vi "SubPanel_DataCollection_Rev11_v4.vi"(0 "DCPowerInformationClusterArray_Input":T6(array[cluster]), 1 "VISAPowerInfoInputArray":T11(array[cluster]), 2 "Run Data SubPanel Input":T10, 3 "RF Block Parameters":T9, 4 "Oscilloscope Info Array":T8(array[cluster]) {"vertical coupling" items=["AC", "DC", "Ground"]}, 6 "New Run?":bool, 7 "error in":errorcluster) -> (10 "data iterating in loop":T2(array[cluster]), 12 "each channel cluster":T2(array[cluster]), 13 "Array of all channels?":dbl[][](array[numeric]), 14 "all channel clusters as a large array":T1(array[cluster]), 16 "data going into the binary file":T3, 20 "DCPowerInformationClusterArray_Output":T6(array[cluster]), 21 "VISAPowerInfoInputOutput":T11(array[cluster]), 22 "Run Data SubPanel Output":T10, 23 "RF Block Parameters Output":T9, 24 "Oscilloscope Info Array Output":T8(array[cluster]) {"vertical coupling" items=["AC", "DC", "Ground"]}, 25 "Reinitialize?":bool, 26 "Data Was Collected?":bool, 27 "error out":errorcluster)   [LabVIEW 2019]
uses:
  Controls/QueueDataControl.ctl
  Controls/DataBlockControl.ctl
  Controls/QueueDataControl_V2.ctl
  <vilib>/Analysis/NI_AALBase.lvlib
  Controls/QueueDataControl_V3.ctl
  <vilib>/Utility/file.llb/Write Delimited Spreadsheet (DBL).vi
  <vilib>/Analysis/1siggen.llb/Ramp Pattern by Delta.vi
  Controls/RFBlockControl.ctl
  <instrlib>/niScope/Controls/niScope vertical coupling.ctl
panel:
  out "supplemental datafile concatenated":i32[](array[numeric])
  out "supplemental datafile array":i32[][](array[numeric])
  out "supplemental datafile":i32[](array[numeric])
  out "datafile in array":T4[][](array[typedef])
  out "datafile in concatenation":T4[](array[typedef])
  out "datafile in loop":T4[](array[typedef])
  out "output cluster 2":T5
  out "Array":dbl[][][](array[numeric])
  out "DCPowerInformationClusterArray_Input 2":T6(array[cluster])
  out "Exiting":bool
  out "output cluster":T5
  out "Full Run Information":string
  out "Ready For Next Run?":bool
  in  "Next Run":bool
  out "Latchup Output Data":dbl[][](array[numeric])
  out "Recording Data":bool
  out "Current 2":waveform(dbl)[](graph)
  out "Voltage 2":waveform(dbl)[](graph)
  out "Current":waveform(dbl)[](graph)
  out "Voltage":waveform(dbl)[](graph)
  in  "End Collecting":bool
  in  "Record Data Toggle":bool
  out "error of collection":errorcluster
  in  "force exit SubVI":bool
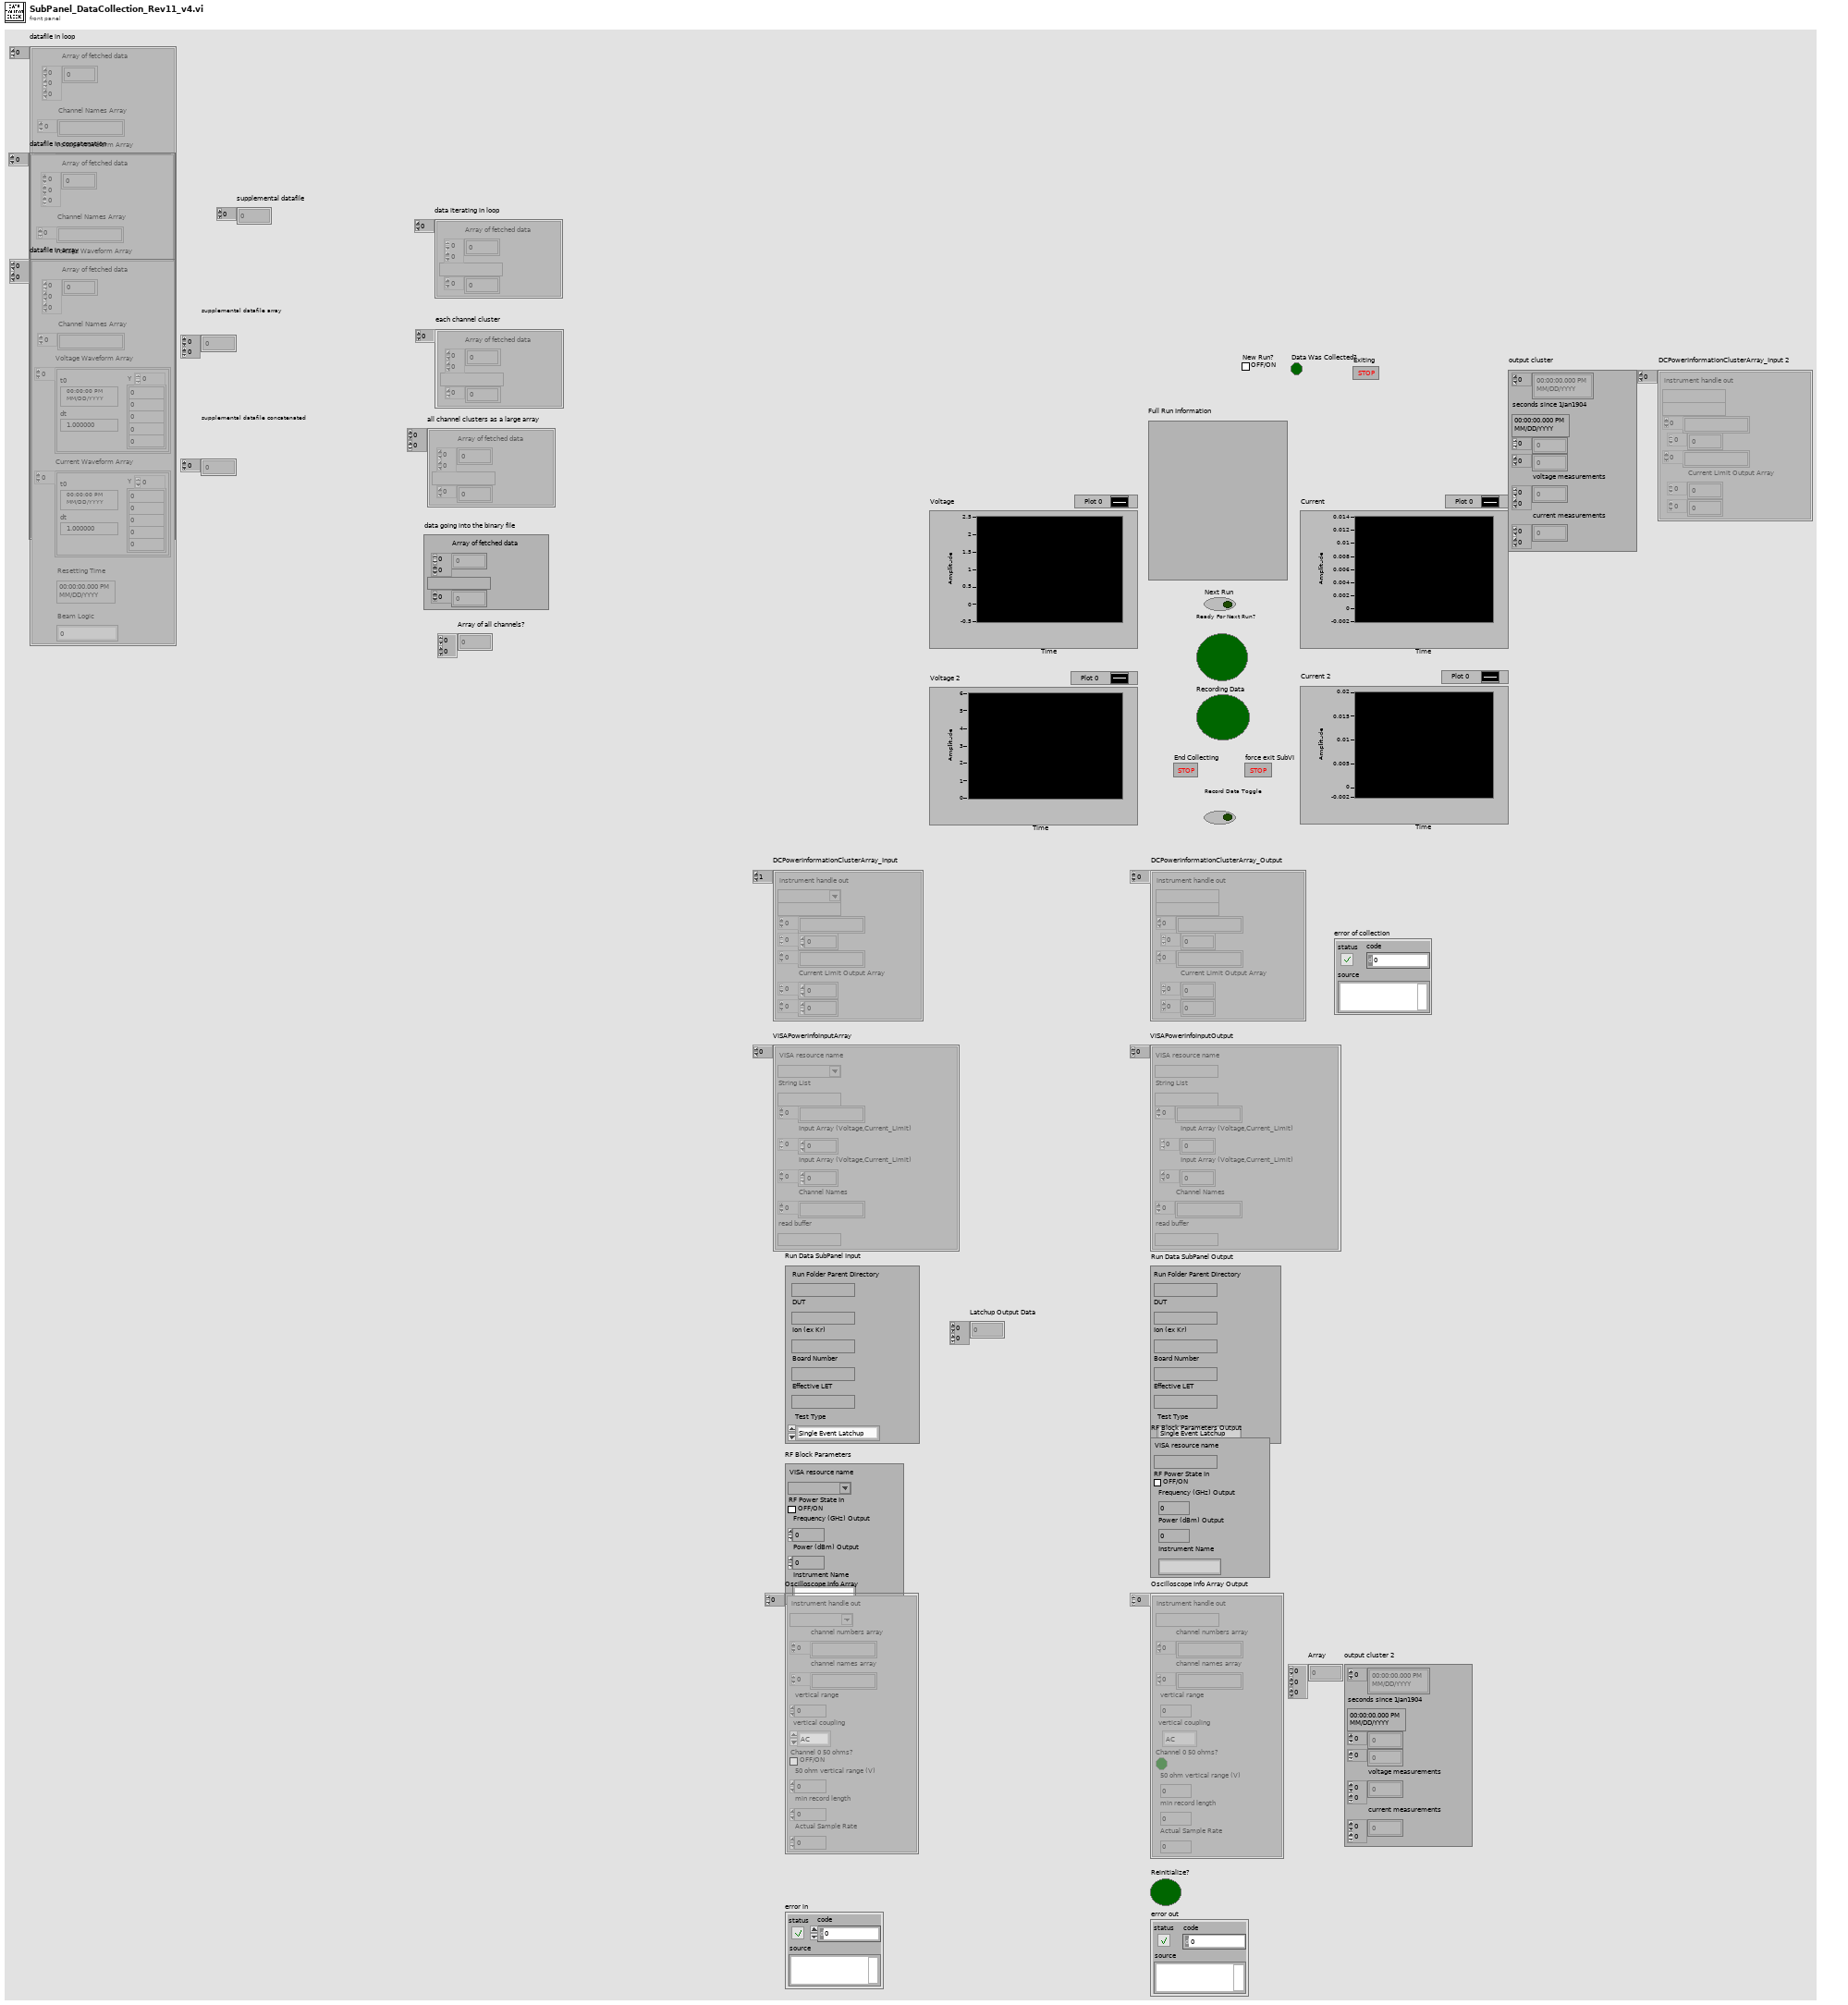
[diagram p1: front panel]
types:
  T1 = cluster{"Array of fetched data":dbl[][], string, i32[]}[][]
  T2 = cluster{"Array of fetched data":dbl[][], string, i32[]}[]
  T3 = cluster{"Array of fetched data":dbl[][], string, i32[]}
  T4 = typedef "QueueDataControl_V3.ctl" = cluster{"Array of fetched data":dbl[][][], "Channel Names Array":string[], "Voltage Waveform Array":waveform(dbl)[], "Current Waveform Array":waveform(dbl)[], "Resetting Time":timestamp, "Beam Logic":dbl}
  T5 = cluster{timestamp[], "seconds since 1Jan1904":timestamp, dbl[], i32[], "voltage measurements":dbl[][], "current measurements":dbl[][]}
  T6 = cluster{"instrument handle out":refnum<k15>, string, string[], dbl[], string[], "Current Limit Output Array":dbl[], dbl[]}[]
  T7 = typedef "niScope vertical coupling.ctl" = i32
  T8 = cluster{"instrument handle out":refnum<k15>, "channel numbers array":string[], "channel names array":string[], "vertical range":dbl, "vertical coupling":T7, "Channel 0 50 ohms?":bool, "50 ohm vertical range (V)":dbl, "min record length":i32, "Actual Sample Rate":dbl}[]
  T9 = typedef "RFBlockControl.ctl" = cluster{"VISA resource name":refnum<visa-resource-name>, "RF Power State In":bool, "Frequency (GHz) Output":dbl, "Power (dBm) Output":dbl, "Instrument Name":string}
  T10 = typedef "DataBlockControl.ctl" = cluster{"Run Folder Parent Directory":path, "DUT":string, "Ion (ex Kr)":string, "Board Number":string, "Effective LET":string, "Test Type":enum16{"Single Event Latchup", "Single Event Transient", "Single Event Upset"}}
  T11 = cluster{"VISA resource name":refnum<visa-resource-name>, "String List":string, string[], "Input Array (Voltage,Current_Limit)":dbl[], "Input Array (Voltage,Current_Limit)":dbl[], "Channel Names":string[], "read buffer":string}[]
  T12 = typedef "QueueDataControl_V2.ctl" = cluster{"Time Stamp Array":timestamp[], "Initial Time":timestamp, "dt measurement array":dbl[], "samples per capture":i32[], "voltage measurements":dbl[][], "current measurements":dbl[][]}
  T13 = cluster{"IVI Refnum out":refnum<k15>, string, "voltage level channel 23":dbl, "Channel Name 23":string, "Current Limit":dbl, "Measure Record dt":dbl, string}[]
  T14 = typedef "QueueDataControl.ctl" = cluster{"Rolling Timer":timestamp, "Initial Time":timestamp, "dt between samples":dbl[], "number of samples per fetch":i32[], "voltage measurements":dbl[][], "current measurements":dbl[][]}
  T15 = enum16{"big-endian, network order", "native, host order", "little-endian"}
  T16 = enum16{"open", "replace", "create", "open or create", "replace or create", "replace or create with confirmation"}
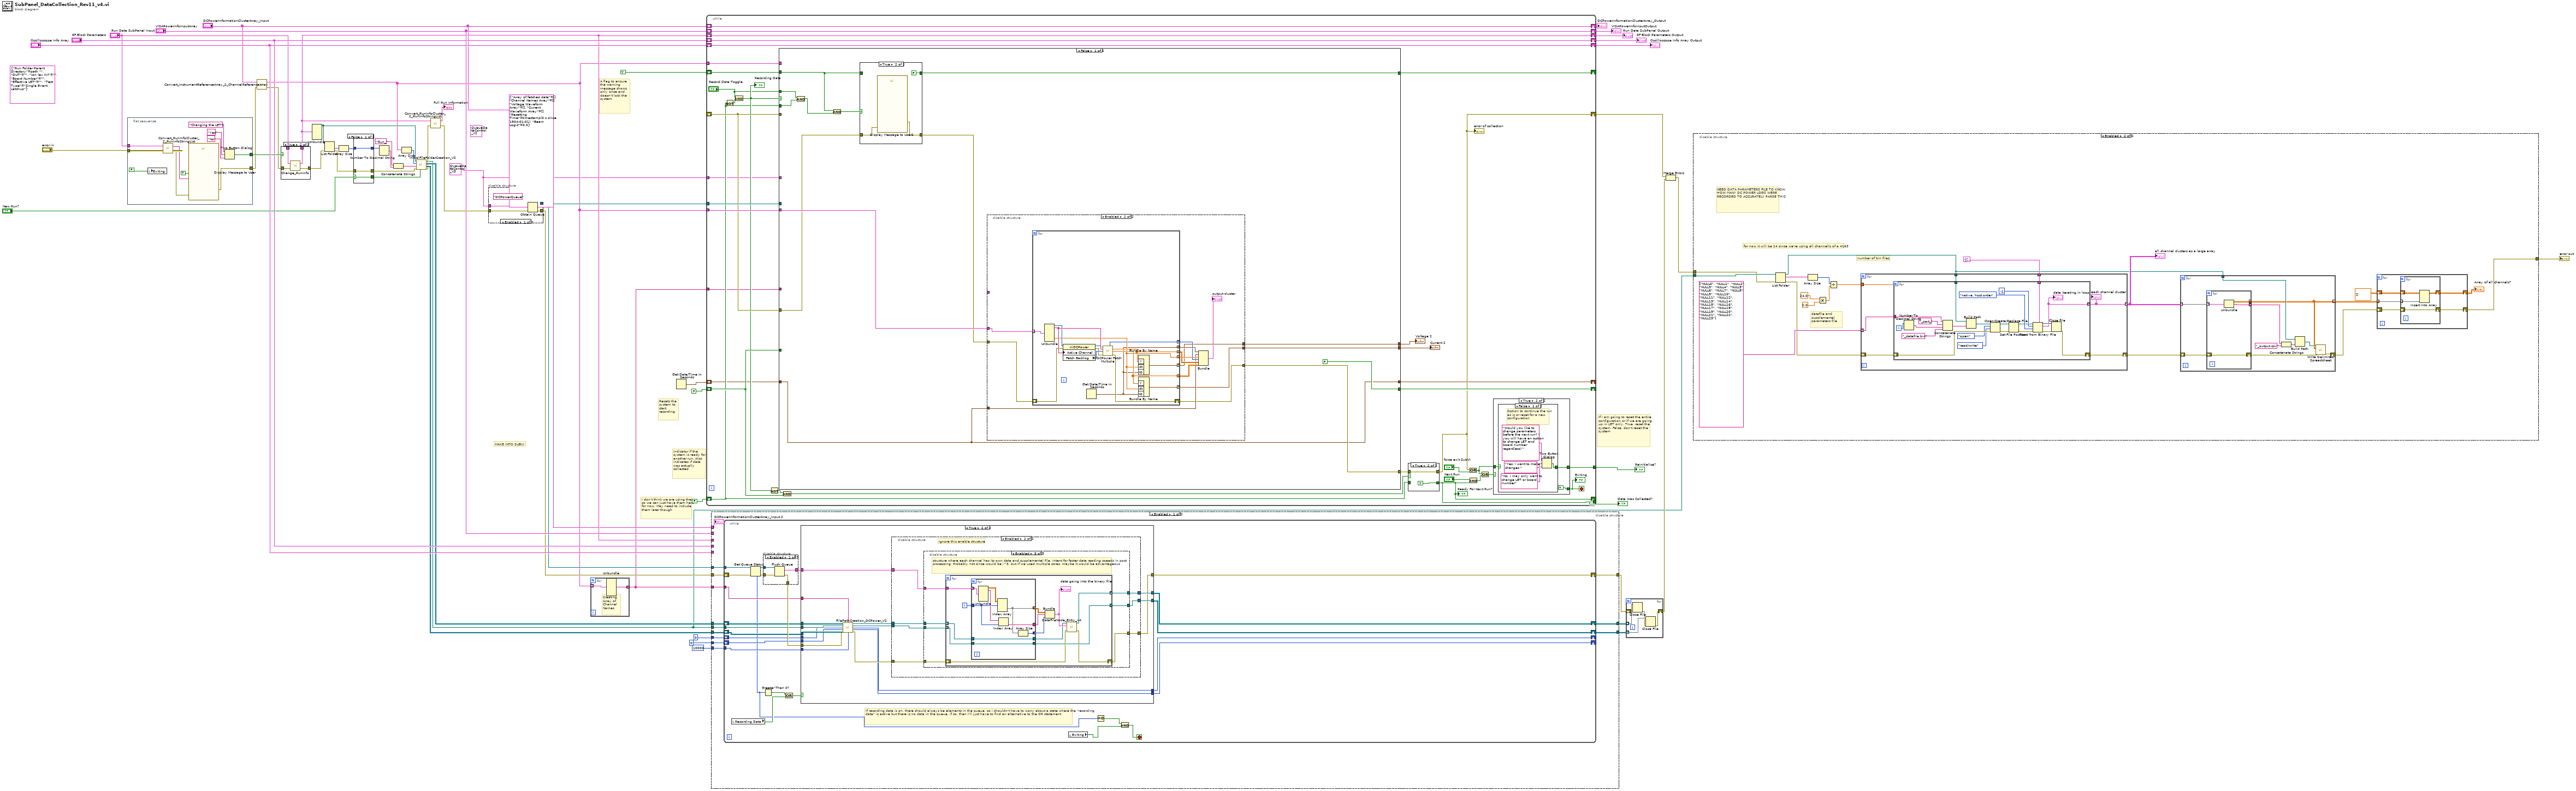
[diagram p0: block diagram]
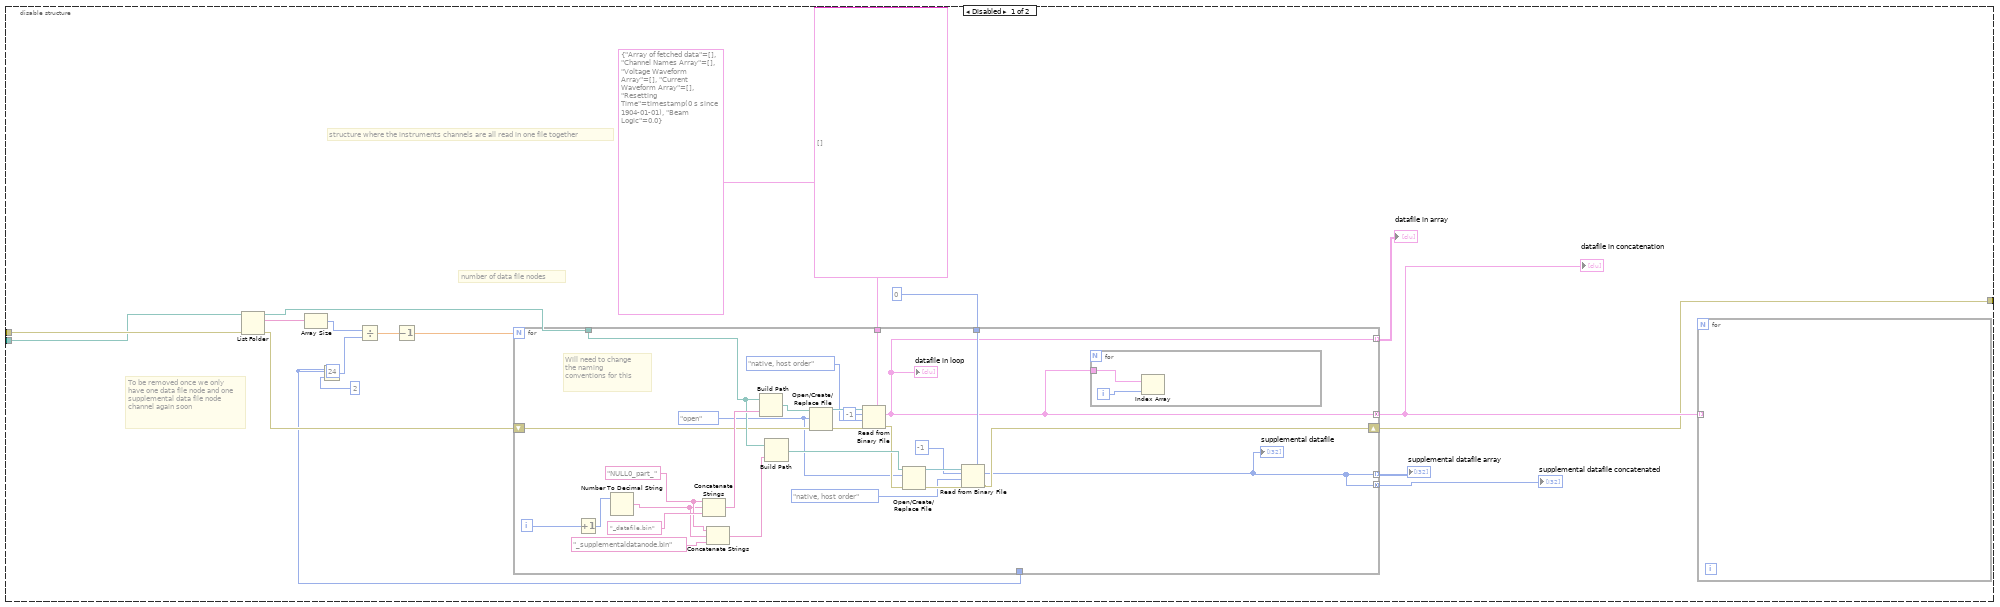
[diagram p2: hidden frame]
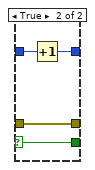
[diagram p3: hidden frame]
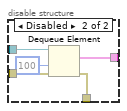
[diagram p6: hidden frame]
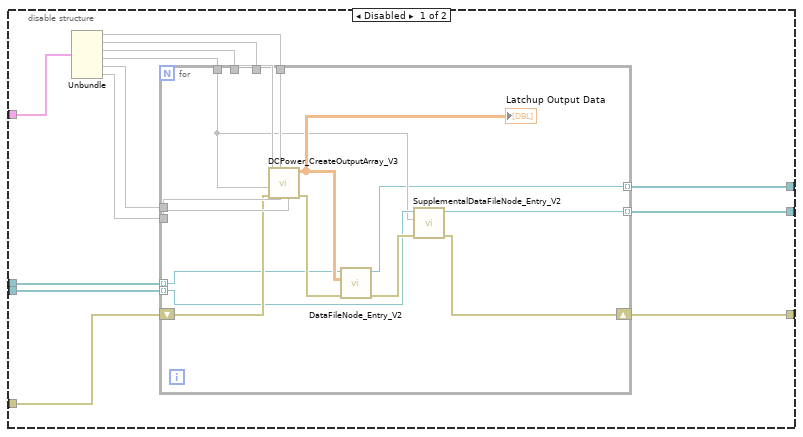
[diagram p8: hidden frame]
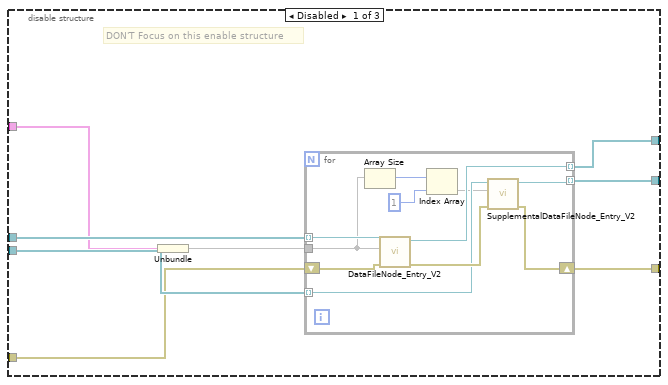
[diagram p9: hidden frame]
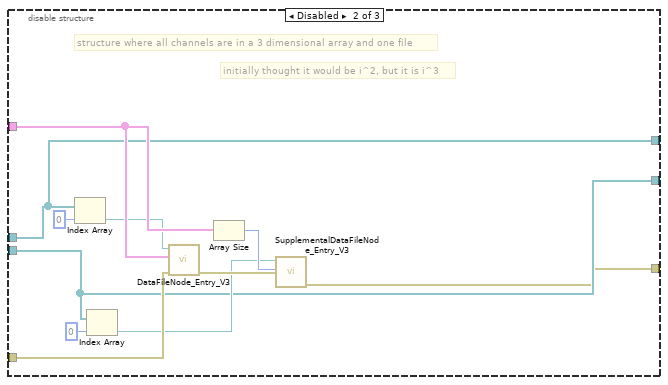
[diagram p10: hidden frame]
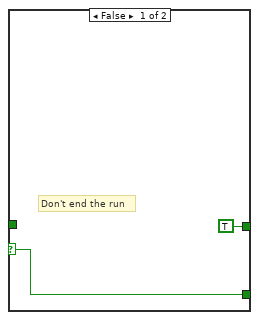
[diagram p12: hidden frame]
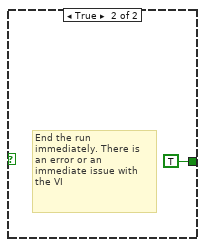
[diagram p13: hidden frame]
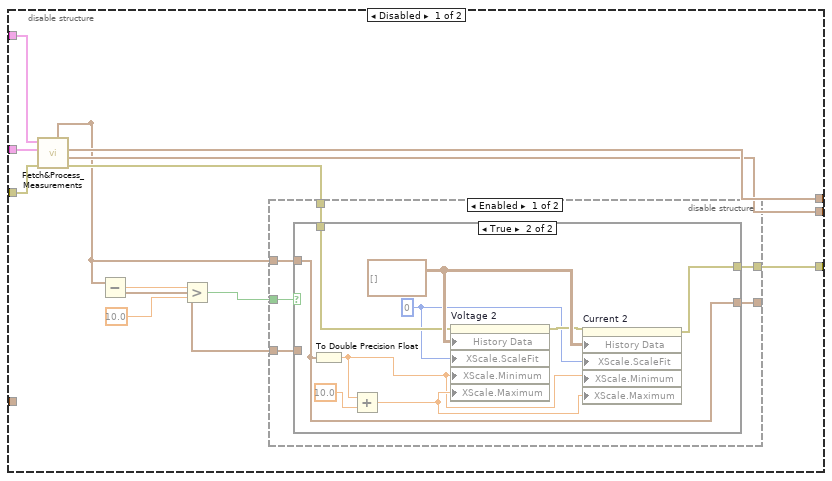
[diagram p15: hidden frame]
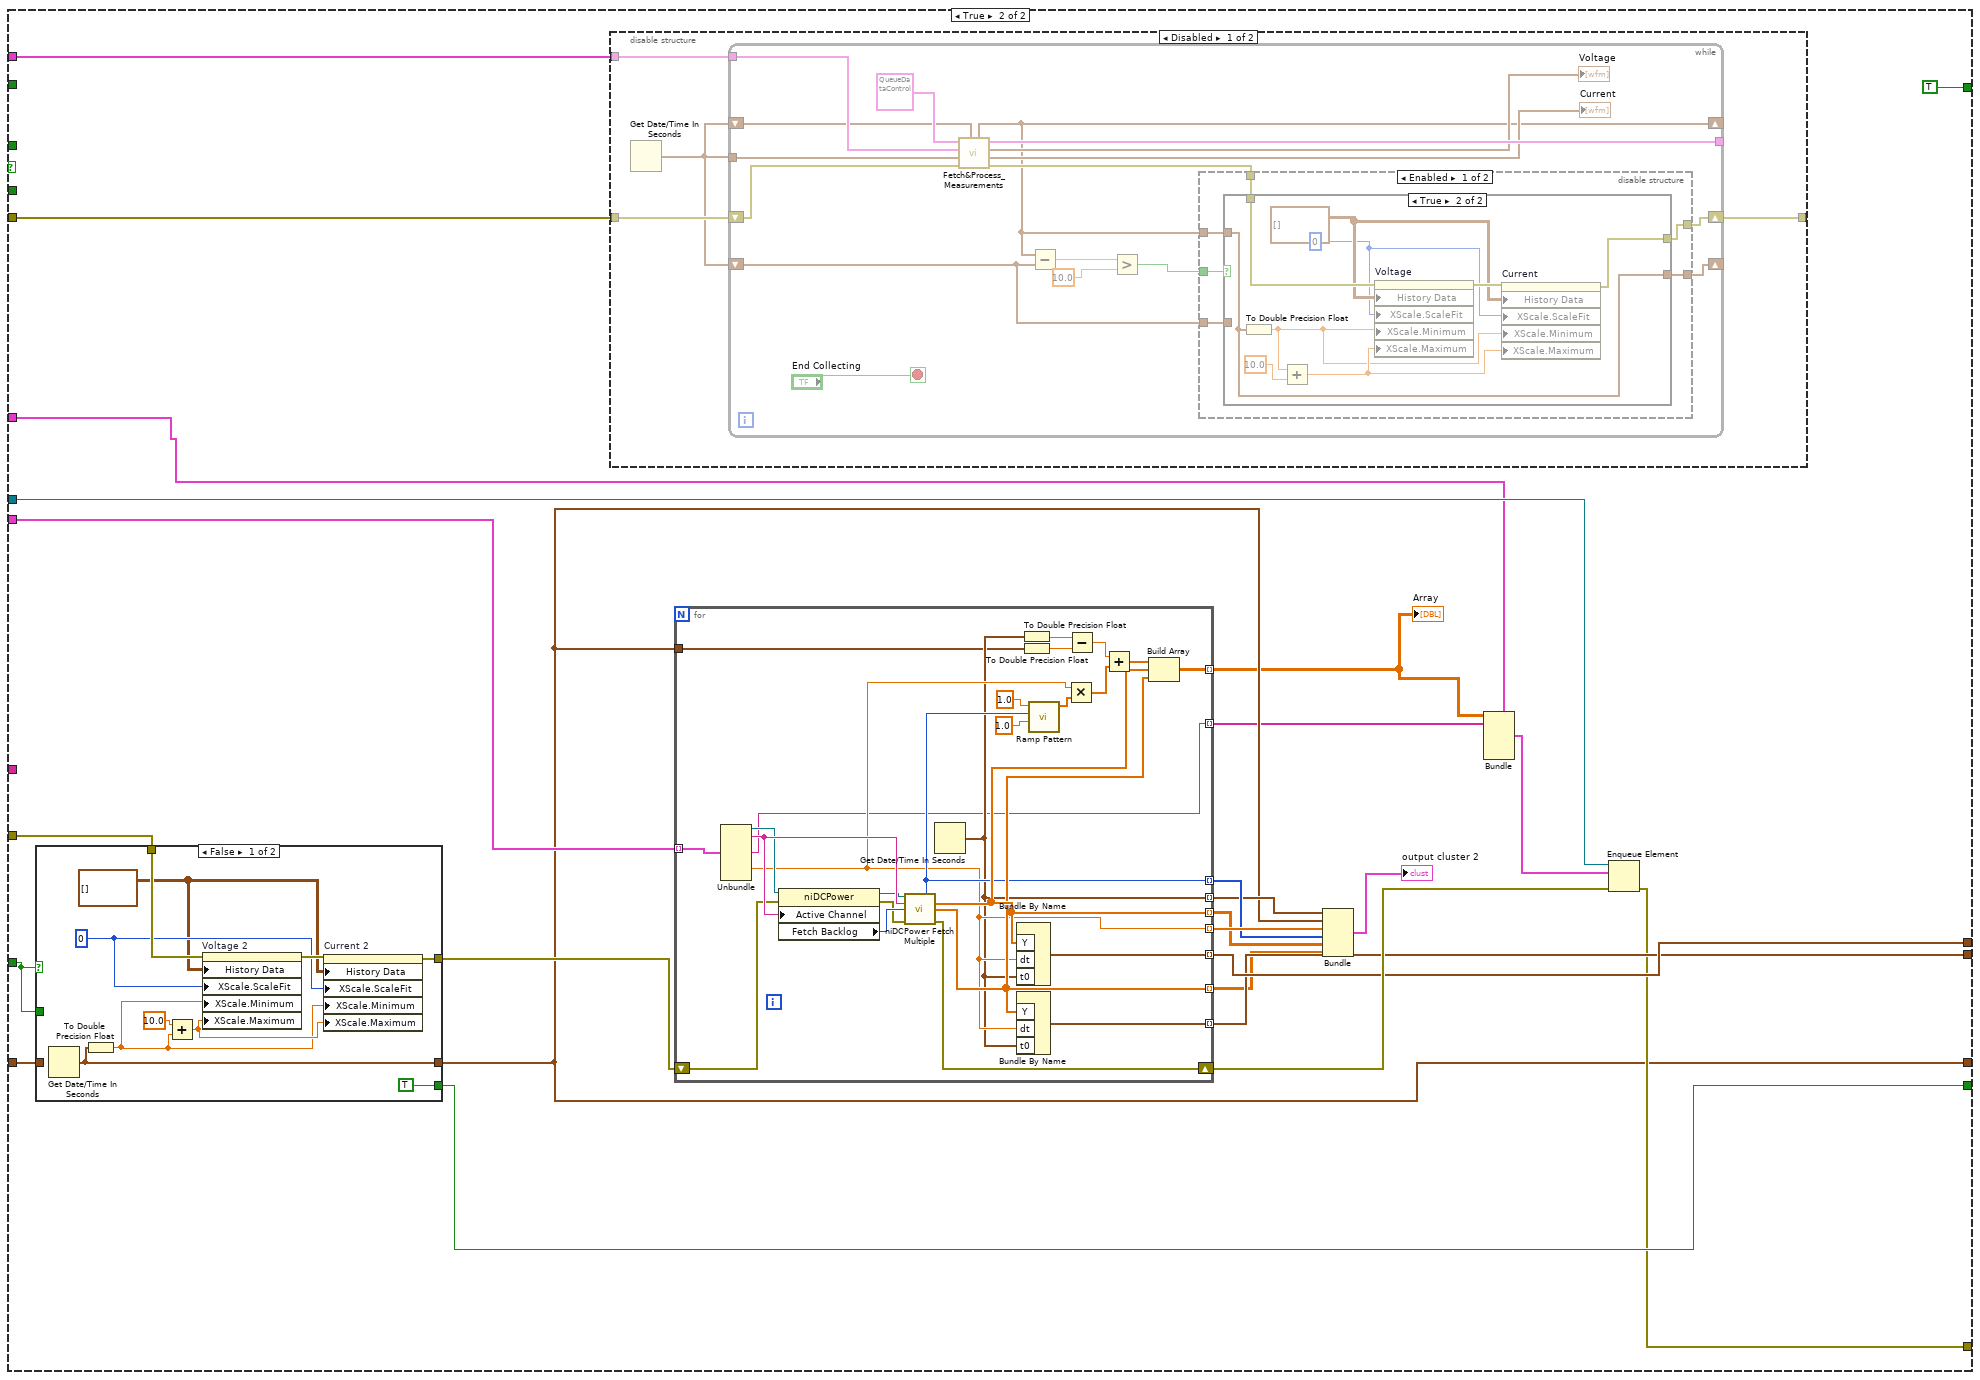
[diagram p19: hidden frame]
diagram:
  w8 = T4 {"Array of fetched data"=[], "Channel Names Array"=[], "Voltage Waveform Array"=[], "Current Waveform Array"=[], "Resetting Time"=timestamp(0 s since 1904-01-01), "Beam Logic"=0.0} ("DCPower Queue Data Double Array Format")
  (unwired) T4 {"Array of fetched data"=[], "Channel Names Array"=[], "Voltage Waveform Array"=[], "Current Waveform Array"=[], "Resetting Time"=timestamp(0 s since 1904-01-01), "Beam Logic"=0.0} ("DCPower Double Array Queue")
  (unwired) T12 {"Time Stamp Array"=[], "Initial Time"=timestamp(0 s since 1904-01-01), "dt measurement array"=[], "samples per capture"=[], "voltage measurements"=[], "current measurements"=[]} ("DCPowerDataQueueControl_V2")
  (unwired) T10 {"Run Folder Parent Directory"=path "", "DUT"="", "Ion (ex Kr)"="", "Board Number"="", "Effective LET"="", "Test Type"=enum."Single Event Latchup"} ("Run Data Configuration")
  # "I don't think we are using these so we can just have them here for now. May need to include them later though"
  # "Indicator if the system is ready for another run. Also indicates if data was actually collected"
  # "Resets the system to start recording"
  # "A flag to ensure the warning message shows only once and doesn't lock the system"
  # "If I am going to reset the entire configuration or if we are going up in LET only. True, reset the system. False, don't reset the system"
  # "MAKE INTO SUBVI"
  n1 = flat-sequence {
    tunnel: [w62] -> w31
    tunnel: "error in" -> [w61]
    tunnel: [w66] -> w40
    tunnel: "Run Data SubPanel Input" -> [w59]
    frame #0 {
      n2 = local write "Exiting"(FALSE ("Forced Exit")) -> ()
      n3 = call "Convert_RunInfoCluster_2_RunInfoStringList.vi"("error in"=w61, "Run Data SubPanel Input"=w59) -> ("error output"=w60:errorcluster, "Run Data Output"=w58:string)
      n4 = call "Display Message to User"("error in (no error)"=w60, "Enable"=TRUE, "Message"=w58) -> ("error out"=w62:errorcluster)  [unwired: 7 in, 1 out]
      n5 = Two Button Dialog(message="Changing the LET?", 1:"No" ("F button name (\"Cancel\")"), 2:"Yes" ("T button name (\"OK\")")) -> (T button?=w66:bool)
    }
  }
  n6 = call "Convert_InstrumentReferenceArray_2_ChannelReferenceArray.vi"("error in (no error)"=w31, "DCPowerInformationClusterArray_Input"="DCPowerInformationClusterArray_Input") -> ("error out"=w29:errorcluster, "DCPowerInformation_byChannel"=w14:T13)
  n7 = case shown="True" w40 {
    tunnel: "Run Data SubPanel Input" -> [w68 w72]
    tunnel: [w68 w71] -> w36
    tunnel: [w67 w70] -> w33
    tunnel: w29 -> [w67 w69]
    frame False {
    }
    frame True {
      n8 = call "Change_RunInfo.vi"("error in (no error)"=w69, "Run Data SubPanel in"=w72) -> ("error out"=w70:errorcluster, "Run Data SubPanel out"=w71:T10)
    }
  }
  n9 = Unbundle(w36) -> ("Run Folder Parent Directory"=w34:path)  [unwired: 5 out]
  n10 = List Folder(path=w34, error in=w33) -> (folder names=w35:string[], error out=w15:errorcluster)  [unwired: 2 in, 2 out]
  n11 = Array Size(array=w35) -> (size(s)=w18:i32)
  n12 = case shown="False" "New Run?" {
    selector: "New Run?" -> [w74 w77]
    tunnel: [w75 w79] -> w19
    tunnel: w18 -> [w75 w78]
    tunnel: [w74 w77] -> w17
    tunnel: [w73 w76] -> w16
    tunnel: w15 -> [w73 w76]
    frame False {
    }
    frame True {
      n13 = Increment(x=w78) -> (x+1=w79:i32)
    }
  }
  n14 = Number To Decimal String(number=w19) -> (decimal integer string=w23:string)  [unwired: 1 in]
  n15 = Concatenate Strings("Run_", w23) -> (w32:string)
  n16 = Array Size(array=w14) -> (size(s)=w13:i32)
  n17 = call "InitialFileFolderCreation_V2.vi"("New Run?"=w17, "error in (no error)"=w16, "Run Number"=w32, "Subfolders&NumChannelsRecorded"=w13, "base path"=w34) -> ("error out"=w12:errorcluster, "SupplementalDataFileReferenceObjectArrayWsubfolders"=w27:refnum<file>[][], "DataFileReferenceObjectArrayWsubfolders"=w28:refnum<file>[][], "created path array"=w2:path[])  [unwired: 3 in]
  n18 = call "Convert_RunInfoCluster_2_RunInfoStringList.vi"("error in"=w12, "Run Data SubPanel Input"=w36) -> ("error output"=w11:errorcluster, "Run Data Output"=→"Full Run Information":string)
  n19 = disable-structure shown="Enabled" {
    disable-tunnel: w11 -> [w83 w85]
    disable-tunnel: [w82 w85] -> w45
    disable-tunnel: [w81 _] -> w46
    disable-tunnel: w8 -> [w80 _]
    frame Enabled {
      n20 = Obtain Queue(name (unnamed)="DCPowerQueue", element data type=w80, error in (no error)=w83) -> (queue out=w81:refnum<queue>, error out=w82:errorcluster)  [unwired: 2 in, 1 out]
    }
    frame Disabled {
    }
  }
  n21 = for {
    tunnel: w14 -> [w87] mode=indexing
    tunnel: [w86] -> w9 mode=indexing
    # "Creating Array of Channel Names"
    n22 = Unbundle(w87) -> ("Channel Name 23"=w86:string)  [unwired: 6 out]
  }
  n23 = Get Date/Time In Seconds() -> (seconds since 1Jan1904=w37:timestamp)
  n24 = while {
    shift-right: [w118] -> w55
    shift-left: "DCPowerInformationClusterArray_Input" -> [w118]
    shift-right: [w122] -> w54
    shift-left: "VISAPowerInfoInputArray" -> [w122]
    shift-right: [w121] -> w53
    shift-left: w36 -> [w121]
    shift-right: [w120] -> w52
    shift-left: "RF Block Parameters" -> [w120]
    shift-right: [w119] -> w51
    shift-left: "Oscilloscope Info Array" -> [w119]
    shift-right: [w102] -> w10
    shift-left: _ -> [w115]
    tunnel: w14 -> [w117]
    tunnel: w14 -> [w116]
    shift-right: [w112] -> _
    shift-left: FALSE -> [w109]
    tunnel: w46 -> [w111]
    shift-right: [w91] -> _
    shift-left: FALSE -> [w96]
    tunnel: [w100] -> w44
    shift-right: [w94] -> _
    shift-left: TRUE ("x .and. y?") -> [w95]
    shift-right: [w92] -> _
    shift-left: w37 -> [w93]
    tunnel: [w91] -> w21
    tunnel: w9 -> [w89]
    tunnel: w8 -> [w88]
    stop <- w90 stop-if-true
    n25 = Not(x=w96) -> (.not. x?=w98:bool)
    n26 = And(x="Record Data Toggle", y=w98) -> (x .and. y?=w99:bool)
    "Recording Data" <- w99
    n27 = Not(x=w99) -> (.not. x?=w110:bool)
    n28 = case shown="False" w99 {
      tunnel: w115 -> [_ w240]
      tunnel: w117 -> [_ w239]
      tunnel: w116 -> [w150 w237]
      tunnel: w115 -> [w145 w235]
      tunnel: [w148 w227] -> w114
      tunnel: [w149 w228] -> w113
      tunnel: w109 -> [_ w232]
      tunnel: [FALSE w233] -> w112
      tunnel: w111 -> [_ w231]
      tunnel: [w146 w226] -> w107
      tunnel: "Record Data Toggle" -> [w142 _]
      tunnel: w96 -> [w143 _]
      tunnel: w95 -> [w138 _]
      tunnel: [w139 TRUE] -> w94
      tunnel: w93 -> [w137 w236]
      tunnel: [w137 w220] -> w92
      tunnel: w89 -> [_ _]
      tunnel: w88 -> [_ w217]
      frame False {
        n29 = And(x=w142, y=w143) -> (x .and. y?=w141:bool)
        n30 = And(x=w138, y=w141) -> (x .and. y?=w140:bool)
        n31 = case shown="True" w140 {
          tunnel: [w212 w214] -> w144
          tunnel: w145 -> [w212 w215]
          tunnel: [w211 FALSE] -> w139
          tunnel: w138 -> [w211 _]
          frame False {
          }
          frame True {
            n32 = call "Display Message to User2"("error in (no error)"=w215) -> ("error out"=w214:errorcluster)  [unwired: 9 in, 1 out]
          }
        }
        n33 = disable-structure shown="Enabled" {
          disable-tunnel: w150 -> [w160 w190]
          disable-tunnel: _ -> [w159 _]
          disable-tunnel: [w155 w188] -> w149
          disable-tunnel: [w154 w187] -> w148
          disable-tunnel: [w152 w186] -> w146
          disable-tunnel: w144 -> [w151 w185]
          disable-tunnel: w137 -> [_ w189]
          frame Disabled {
            n34 = call "Fetch&Process_Measurements.vi"("error in (no error)"=w151, "DCPowerInformation_byChannel"=w160, "Queue Data Parameters in"=w159) -> ("error out"=w161:errorcluster, "Current Measurement"=w154:waveform(dbl)[], "Voltage Measurement"=w155:waveform(dbl)[], "Rolling Timer Output"=w153:timestamp, "Rolling Timer Input"=w158:timestamp)  [unwired: 3 in, 1 out]
            n35 = Subtract(x=w153, y=w156) -> (x-y=w163:dbl)
            n36 = Greater?(x=w163, y=10.0) -> (0:w162:bool)
            n37 = disable-structure shown="Enabled" {
              disable-tunnel: w162 -> [w170 _]
              disable-tunnel: w161 -> [w169 w183]
              disable-tunnel: [w168 w183] -> w152
              disable-tunnel: [w167 w182] -> w157
              disable-tunnel: w153 -> [w166 w182]
              disable-tunnel: [w165 _] -> w156
              frame Enabled {
                n38 = case shown="True" w170 {
                  tunnel: w169 -> [w172 w178]
                  tunnel: [w172 w176] -> w168
                  tunnel: [w171 w180] -> w167
                  tunnel: w166 -> [_ w180]
                  tunnel: w165 -> [w171 _]
                  frame False {
                  }
                  frame True {
                    w175 = u8 0 ("X Scale.Scale Fit")
                    w179 = waveform(dbl)[][] [] ("History Data")
                    n39 = To Double Precision Float(number=w180) -> (double precision float=w173:dbl)
                    n40 = Add(x=w173, y=10.0) -> (x+y=w174:dbl)
                    n41 = property on="Voltage 2" class="WFChart (strict)"(error in=w178, "History Data"=w179, "XScale.ScaleFit"=w175, "XScale.Minimum"=w173, "XScale.Maximum"=w174) -> (error out=w177:errorcluster)  [unwired: 1 in, 1 out]
                    n42 = property on="Current 2" class="WFChart (strict)"(error in=w177, "History Data"=w179, "XScale.ScaleFit"=w175, "XScale.Minimum"=w173, "XScale.Maximum"=w174) -> (error out=w176:errorcluster)  [unwired: 1 in, 1 out]
                  }
                }
              }
              frame Disabled {
              }
            }
          }
          frame Enabled {
            n43 = for {
              tunnel: w190 -> [w210] mode=indexing
              tunnel: [w203] -> w188 mode=indexing
              tunnel: [w202] -> w187 mode=indexing
              tunnel: [w197] -> w192 mode=indexing
              tunnel: [w201] -> w194 mode=indexing
              tunnel: [w200] -> w193 mode=indexing
              tunnel: [w196] -> w195 mode=indexing
              tunnel: [w198] -> w191 mode=indexing
              shift-right: [w199] -> w186
              shift-left: w185 -> [w207]
              n44 = Unbundle(w210) -> ("IVI Refnum out"=w206:refnum<k15>, w209:string, "Measure Record dt"=w198:dbl)  [unwired: 4 out]
              n45 = property class="niDCPower"(reference=w206, error in=w207, "Active Channel"=w209) -> (reference out=w205:refnum<k15>, error out=w204:errorcluster, "Fetch Backlog"=w208:i32)
              n46 = Get Date/Time In Seconds() -> (seconds since 1Jan1904=w196:timestamp)
              n47 = call <instrlib>:"niDCPower Fetch Multiple.vi"("instrument handle"=w205, "channel name"=w209, "count (1)"=w208, "error in (no error)"=w204) -> ("actual count"=w197:i32, "voltage measurements"=w200:dbl[], "current measurements"=w201:dbl[], "error out"=w199:errorcluster)  [unwired: 6 in, 2 out]
              n48 = Bundle By Name("Y"=w200, "dt"=w198, "t0"=w196) -> (w203:waveform(dbl))  [unwired: 1 out]
              n49 = Bundle By Name("Y"=w201, "dt"=w198, "t0"=w196) -> (w202:waveform(dbl))  [unwired: 1 out]
            }
            n50 = Bundle(w195, "seconds since 1Jan1904"=w189, w191, w192, "voltage measurements"=w193, "current measurements"=w194) -> (→"output cluster":T5)  [unwired: 1 in]
          }
        }
      }
      frame True {
        n51 = case shown="False" w232 {
          tunnel: [w271 w279] -> w220
          tunnel: w236 -> [_ w279]
          tunnel: w235 -> [w276 w278]
          tunnel: [w274 w278] -> w234
          tunnel: [TRUE w277] -> w233
          tunnel: w232 -> [_ w277]
          frame False {
            w267 = waveform(dbl)[][] [] ("History Data")
            w272 = u8 0 ("X Scale.Scale Fit")
            n52 = Get Date/Time In Seconds() -> (seconds since 1Jan1904=w271:timestamp)
            n53 = To Double Precision Float(number=w271) -> (double precision float=w268:dbl)
            n54 = Add(x=10.0 ("y"), y=w268) -> (x+y=w270:dbl)
            n55 = property on="Voltage 2" class="WFChart (strict)"(error in=w276, "History Data"=w267, "XScale.ScaleFit"=w272, "XScale.Minimum"=w268, "XScale.Maximum"=w270) -> (error out=w275:errorcluster)  [unwired: 1 in, 1 out]
            n56 = property on="Current 2" class="WFChart (strict)"(error in=w275, "History Data"=w267, "XScale.ScaleFit"=w272, "XScale.Minimum"=w268, "XScale.Maximum"=w270) -> (error out=w274:errorcluster)  [unwired: 1 in, 1 out]
          }
          frame True {
          }
        }
        n57 = disable-structure shown="Disabled" {
          disable-tunnel: w240 -> [w283 _]
          disable-tunnel: w239 -> [w282 _]
          disable-tunnel: [w281 errorcluster {"status"=FALSE, "code"=0, "source"=""} ("error out")] -> _
          frame Disabled {
            n58 = Get Date/Time In Seconds() -> (seconds since 1Jan1904=w280:timestamp)
            n59 = while {
              shift-right: [w287] -> w281
              shift-left: w283 -> [w298]
              tunnel: w282 -> [w299]
              tunnel: w280 -> [w295]
              shift-right: [w285] -> _
              shift-left: w280 -> [w296]
              tunnel: [w294] -> _
              shift-right: [w286] -> _
              shift-left: w280 -> [w284]
              stop <- "End Collecting" stop-if-true
              n60 = call "Fetch&Process_Measurements.vi"("Rolling Timer Input"=w296, "error in (no error)"=w298, "Initial Time"=w295, "DCPowerInformation_byChannel"=w299, "Queue Data Parameters in"=T14 {"Rolling Timer"=timestamp(0 s since 1904-01-01), "Initial Time"=timestamp(0 s since 1904-01-01), "dt between samples"=[], "number of samples per fetch"=[], "voltage measurements"=[], "current measurements"=[]} ("Queue Data Parameters")) -> ("error out"=w288:errorcluster, "Current Measurement"=→"Current":waveform(dbl)[], "Voltage Measurement"=→"Voltage":waveform(dbl)[], "Queue Data Parameters out"=w294:T14, "Rolling Timer Output"=w285:timestamp)  [unwired: 2 in]
              n61 = Subtract(x=w285, y=w284) -> (x-y=w290:dbl)
              n62 = Greater?(x=w290, y=10.0) -> (0:w289:bool)
              n63 = disable-structure shown="Enabled" {
                disable-tunnel: w289 -> [w306 _]
                disable-tunnel: w288 -> [w305 w319]
                disable-tunnel: [w304 w319] -> w287
                disable-tunnel: [w303 w318] -> w286
                disable-tunnel: w285 -> [w302 w318]
                disable-tunnel: w284 -> [w301 _]
                frame Enabled {
                  n64 = case shown="True" w306 {
                    tunnel: w305 -> [w308 w317]
                    tunnel: [w308 w315] -> w304
                    tunnel: [w307 w309] -> w303
                    tunnel: w302 -> [_ w309]
                    tunnel: w301 -> [w307 _]
                    frame False {
                    }
                    frame True {
                      w312 = u8 0 ("X Scale.Scale Fit")
                      w313 = waveform(dbl)[][] [] ("History Data")
                      n65 = To Double Precision Float(number=w309) -> (double precision float=w310:dbl)
                      n66 = Add(x=w310, y=10.0) -> (x+y=w311:dbl)
                      n67 = property on="Voltage" class="WFChart (strict)"(error in=w317, "History Data"=w313, "XScale.ScaleFit"=w312, "XScale.Minimum"=w310, "XScale.Maximum"=w311) -> (error out=w316:errorcluster)  [unwired: 1 in, 1 out]
                      n68 = property on="Current" class="WFChart (strict)"(error in=w316, "History Data"=w313, "XScale.ScaleFit"=w312, "XScale.Minimum"=w310, "XScale.Maximum"=w311) -> (error out=w315:errorcluster)  [unwired: 1 in, 1 out]
                    }
                  }
                }
                frame Disabled {
                }
              }
            }
          }
          frame Enabled {
          }
        }
        n69 = for {
          tunnel: w237 -> [w266] mode=indexing
          tunnel: [w259] -> w228 mode=indexing
          tunnel: [w258] -> w227 mode=indexing
          tunnel: [w246] -> w224 mode=indexing
          tunnel: [w247] -> w222 mode=indexing
          tunnel: [w248] -> w223 mode=indexing
          tunnel: [w244] -> w221 mode=indexing
          tunnel: [w245] -> w225 mode=indexing
          shift-right: [w257] -> w230
          shift-left: w234 -> [w263]
          tunnel: w220 -> [w243]
          tunnel: [w242] -> w219 mode=indexing
          tunnel: [w241] -> w218 mode=indexing
          n70 = Unbundle(w266) -> ("IVI Refnum out"=w262:refnum<k15>, w265:string, "Channel Name 23"=w241:string, "Measure Record dt"=w245:dbl)  [unwired: 3 out]
          n71 = property class="niDCPower"(reference=w262, error in=w263, "Active Channel"=w265) -> (reference out=w261:refnum<k15>, error out=w260:errorcluster, "Fetch Backlog"=w264:i32)
          n72 = call <instrlib>:"niDCPower Fetch Multiple.vi"("instrument handle"=w261, "channel name"=w265, "count (1)"=w264, "error in (no error)"=w260) -> ("actual count"=w246:i32, "voltage measurements"=w248:dbl[], "current measurements"=w247:dbl[], "error out"=w257:errorcluster)  [unwired: 6 in, 2 out]
          n73 = Get Date/Time In Seconds() -> (seconds since 1Jan1904=w244:timestamp)
          n74 = Bundle By Name("Y"=w248, "dt"=w245, "t0"=w244) -> (w259:waveform(dbl))  [unwired: 1 out]
          n75 = Bundle By Name("Y"=w247, "dt"=w245, "t0"=w244) -> (w258:waveform(dbl))  [unwired: 1 out]
          n76 = To Double Precision Float(number=w244) -> (double precision float=w254:dbl)
          n77 = To Double Precision Float(number=w243) -> (double precision float=w253:dbl)
          n78 = call-poly <vilib>:"Ramp Pattern.vi"("start"=1.0, "end"=w246, "delta"=1.0) -> ("Ramp Pattern"=w250:dbl[])  [unwired: 6 in, 2 out]
          n79 = Multiply(x=w245, y=w250) -> (x*y=w249:dbl[])
          n80 = Subtract(x=w254, y=w253) -> (x-y=w251:dbl)
          n81 = Add(x=w251, y=w249) -> (x+y=w256:dbl[])
          n82 = Build Array(w256, w248, w247) -> (w242:dbl[][])
        }
        "Array" <- w219
        n83 = Bundle(w221, "seconds since 1Jan1904"=w220, w225, w224, "voltage measurements"=w223, "current measurements"=w222) -> (→"output cluster 2":T5)  [unwired: 1 in]
        n84 = Bundle(cluster=w217, "Array of fetched data"=w219, "Channel Names Array"=w218) -> (w216:T4)  [unwired: 4 in]
        n85 = Enqueue Element(queue=w231, element=w216, error in (no error)=w230) -> (error out=w226:errorcluster)  [unwired: 1 in, 2 out]
      }
    }
    "Voltage 2" <- w113
    "Current 2" <- w114
    n86 = And(x=w110, y=w109) -> (x .and. y?=w108:bool)
    n87 = case shown="True" w108 {
      tunnel: w107 -> [w133 w135]
      tunnel: [w134 TRUE] -> w91
      tunnel: w96 -> [w134 _]
      tunnel: [w133 w135] -> w102
      frame False {
      }
      frame True {
      }
    }
    "error of collection" <- w102
    "Ready For Next Run?" <- w91
    n88 = Or(x=w102, y="force exit SubVI") -> (x .or. y?=w104:bool)
    n89 = And(x="Next Run", y=w91) -> (x .and. y?=w106:bool)
    n90 = Or(x=w104, y=w106) -> (x .or. y?=w105:bool)
    n91 = case shown="True" w105 {
      selector: w105 -> [w124 _]
      tunnel: w104 -> [_ w127]
      tunnel: [w124 TRUE] -> w90
      tunnel: [TRUE ("T button?") w125] -> w100
      frame False {
        # "Don't end the run"
      }
      frame True {
        n92 = case shown="False" w127 {
          tunnel: [w128 TRUE] -> w125
          frame False {
            # "Option to continue the run as is or reset for a new configuration"
            n93 = Two Button Dialog(message="Would you like to change parameters before the next run? ( you will have an option to change LET and board number regardless) ", 1:"No, I may only want to change LET or board number" ("F button name (\"Cancel\")"), 2:"Yes, I want to make changes " ("T button name (\"OK\")")) -> (T button?=w128:bool)
          }
          frame True {
            # "End the run immediately. There is an error or an immediate issue with the VI"
          }
        }
      }
    }
    "Exiting" <- w90
  }
  "DCPowerInformationClusterArray_Output" <- w55
  "VISAPowerInfoInputOutput" <- w54
  "Run Data SubPanel Output" <- w53
  "RF Block Parameters Output" <- w52
  "Oscilloscope Info Array Output" <- w51
  "Reinitialize?" <- w44
  "Data Was Collected?" <- w21
  n94 = disable-structure shown="Enabled" {
    disable-tunnel: "DCPowerInformationClusterArray_Input" -> [w324 _]
    disable-tunnel: "VISAPowerInfoInputArray" -> [_ _]
    disable-tunnel: w36 -> [_ _]
    disable-tunnel: "RF Block Parameters" -> [_ _]
    disable-tunnel: "Oscilloscope Info Array" -> [_ _]
    disable-tunnel: w46 -> [w333 _]
    disable-tunnel: w45 -> [w332 _]
    disable-tunnel: w9 -> [w331 _]
    disable-tunnel: w2 -> [w330 _]
    disable-tunnel: w28 -> [w329 _]
    disable-tunnel: w27 -> [w328 _]
    disable-tunnel: 0 ("binary file indexor in") -> [w327 _]
    disable-tunnel: 0 ("binary file indexor in") -> [w326 _]
    disable-tunnel: 10000 ("binary file indexor in") -> [w325 _]
    disable-tunnel: [w323 _] -> w5
    disable-tunnel: [w322 _] -> w7
    disable-tunnel: [w321 _] -> w6
    frame Enabled {
      n95 = while {
        tunnel: w333 -> [w351]
        shift-right: [w338] -> w323
        shift-left: w332 -> [w350]
        tunnel: w330 -> [w347]
        shift-right: [w340] -> w322
        shift-left: w329 -> [w348]
        shift-right: [w339] -> w321
        shift-left: w328 -> [w346]
        shift-right: [w342] -> _
        shift-left: w327 -> [w345]
        shift-right: [w341] -> _
        shift-left: w326 -> [w344]
        tunnel: w325 -> [w343]
        tunnel: w331 -> [w349]
        stop <- w334 stop-if-true
        # "If recording data is on, there should always be elements in the queue, so I shouldn't have to worry about a state where the \"recording data\" is active but there is no data in the queue, if so, then I'll just have to find an alternative to the OR statement"
        n96 = local read "Recording Data"() -> (w356:bool)
        n97 = Get Queue Status(queue=w351, error in (no error)=w350) -> (queue out=w353:refnum<queue>, error out=w354:errorcluster, # elements in queue=w337:i32)  [unwired: 1 in, 5 out]
        n98 = disable-structure shown="Enabled" {
          disable-tunnel: [w362 w364] -> w355
          disable-tunnel: w354 -> [w361 w366]
          disable-tunnel: w353 -> [w360 w367]
          disable-tunnel: [w359 w363] -> w352
          frame Enabled {
            n99 = Flush Queue(queue=w360, error in (no error)=w361) -> (remaining elements=w359:T4[], error out=w362:errorcluster)  [unwired: 1 out]
          }
          frame Disabled {
            n100 = Dequeue Element(queue=w367, timeout in ms (-1)=100, error in (no error)=w366) -> (element=w363:T4, error out=w364:errorcluster)  [unwired: 2 out]
          }
        }
        n101 = Greater Than 0?(x=w337) -> (x > 0?=w357:bool)
        n102 = Or(x=w357, y=w356) -> (x .or. y?=w358:bool)
        n103 = case shown="True" w358 {
          tunnel: w352 -> [_ w389]
          tunnel: w355 -> [w370 w382]
          tunnel: w349 -> [_ w388]
          tunnel: w348 -> [w371 w387]
          tunnel: w347 -> [_ w386]
          tunnel: w346 -> [w372 w385]
          tunnel: w345 -> [w369 w384]
          tunnel: w344 -> [w368 w381]
          tunnel: w343 -> [_ w380]
          tunnel: [w369 w379] -> w342
          tunnel: [w368 w378] -> w341
          tunnel: [w371 w375] -> w340
          tunnel: [w372 w374] -> w339
          tunnel: [w370 w373] -> w338
          frame False {
          }
          frame True {
            n104 = call "FilePathCreation_DCPower_V2.vi"("binary file input reference array 1"=w387, "Channel Name Input array"=w388, "data output directory folder"=w386, "binary file indexor in"=w384, "Reset counter in"=w381, "error in (no error)"=w382, "binary file input reference array 2"=w385, "reset threshold"=w380) -> ("binary file output reference array"=w377:refnum<file>[], "binary file output reference array 2"=w376:refnum<file>[], "binary file indexor out"=w379:i32, "reset counter out"=w378:i32, "error out"=w383:errorcluster)  [unwired: 3 in]
            n105 = disable-structure shown="Enabled" {
              disable-tunnel: w389 -> [w402 w418]
              disable-tunnel: w383 -> [w401 w422]
              disable-tunnel: w377 -> [w400 w424]
              disable-tunnel: w376 -> [w399 w423]
              disable-tunnel: [w398 w421] -> w375
              disable-tunnel: [w397 w420] -> w374
              disable-tunnel: [w396 w419] -> w373
              frame Disabled {
                n106 = Unbundle(w402) -> (w390, w391, w395, w394, w393, w392)
                n107 = for {
                  tunnel: w395 -> [w415]
                  tunnel: w394 -> [w405]
                  tunnel: w393 -> [w414]
                  tunnel: w392 -> [w413]
                  tunnel: w391 -> [w416]
                  tunnel: w390 -> [w417]
                  shift-right: [w407] -> w396
                  shift-left: w401 -> [w412]
                  tunnel: w400 -> [w409] mode=indexing
                  tunnel: w399 -> [w406] mode=indexing
                  tunnel: [w404] -> w398 mode=indexing
                  tunnel: [w403] -> w397 mode=indexing
                  n108 = call "DCPower_CreateOutputArray_V3.vi"("current measurements"=w413, "voltage measurements"=w414, "Time Stamp Array"=w417, "error in"=w412, "actual count"=w405, "Measure Record dt"=w415, "Initial Time"=w416) -> ("error out"=w411:errorcluster, "Data Output Array"=w410:dbl[][])  [unwired: 3 in]
                  "Latchup Output Data" <- w410
                  n109 = call "DataFileNode_Entry_V2.vi"("error in (no error)"=w411, "Data Output Array"=w410, "Byte Stream File in"=w409) -> ("error out"=w408:errorcluster, "Byte Stream File out"=w404:refnum<file>)  [unwired: 7 in]
                  n110 = call "SupplementalDataFileNode_Entry_V2.vi"("error in (no error)"=w408, "actual count"=w405, "Byte Stream File in"=w406) -> ("error out"=w407:errorcluster, "Byte Stream File out"=w403:refnum<file>)  [unwired: 7 in]
                }
              }
              frame Enabled {
                # "Ignore this enable structure"
                n111 = disable-structure shown="Enabled" {
                  disable-tunnel: w424 -> [w432 w446 w461]
                  disable-tunnel: w423 -> [w431 w445 w460]
                  disable-tunnel: w422 -> [w430 w454 w458]
                  disable-tunnel: [w429 w446 w456] -> w421
                  disable-tunnel: [w428 w445 w455] -> w420
                  disable-tunnel: [w427 w444 w459] -> w419
                  disable-tunnel: w418 -> [w426 w451 w457]
                  frame Disabled {
                    # "DON'T Focus on this enable structure"
                    n112 = Unbundle(w426) -> (w425)
                    n113 = for {
                      tunnel: w425 -> [w440]
                      tunnel: w432 -> [w442] mode=indexing
                      tunnel: w431 -> [w441] mode=indexing
                      tunnel: [w438] -> w429 mode=indexing
                      tunnel: [w437] -> w428 mode=indexing
                      shift-right: [w436] -> w427
                      shift-left: w430 -> [w439]
                      n114 = Array Size(array=w440) -> (size(s)=w435:i32)
                      n115 = call "DataFileNode_Entry_V2.vi"("error in (no error)"=w439, "Data Output Array"=w440, "Byte Stream File in"=w442) -> ("error out"=w443:errorcluster, "Byte Stream File out"=w438:refnum<file>)  [unwired: 7 in]
                      n116 = Index Array(array=w435, index=1) -> (element=w433)
                      n117 = call "SupplementalDataFileNode_Entry_V2.vi"("error in (no error)"=w443, "actual count"=w433, "Byte Stream File in"=w441) -> ("error out"=w436:errorcluster, "Byte Stream File out"=w437:refnum<file>)  [unwired: 7 in]
                    }
                  }
                  frame Disabled {
                    # "initially thought it would be i^2, but it is i^3"
                    # "structure where all channels are in a 3 dimensional array and one file"
                    n118 = Index Array(array=w446, index=0) -> (element=w447:refnum<file>)
                    n119 = Index Array(array=w445, index=0) -> (element=w448:refnum<file>)
                    n120 = call "DataFileNode_Entry_V3.vi"("error in (no error)"=w454, "remaining elements"=w451, "Byte Stream File in"=w447) -> ("error out"=w453:errorcluster)  [unwired: 7 in, 1 out]
                    n121 = Array Size(array=w451) -> (size(s)=w452:i32)
                    n122 = call "SupplementalDataFileNode_Entry_V3.vi"("error in (no error)"=w453, "actual count"=w452, "Byte Stream File in"=w448) -> ("error out"=w444:errorcluster)  [unwired: 7 in, 1 out]
                  }
                  frame Enabled {
                    # "structure where each channel has its own data and supplemental file. Intent for faster data reading speeds in post processing. Probably not since would be i^3, but if we used multiple cores, maybe it would be advantageous"
                    n123 = for {
                      tunnel: w461 -> [w469] mode=indexing
                      tunnel: w460 -> [w470] mode=indexing
                      shift-right: [w462] -> w459
                      shift-left: w458 -> [w465]
                      tunnel: w457 -> [w474]
                      tunnel: [w464] -> w456 mode=indexing
                      tunnel: [w463] -> w455 mode=indexing
                      i -> [w473]
                      n124 = for {
                        tunnel: w474 -> [w483] mode=indexing
                        tunnel: w473 -> [w480]
                        tunnel: [w476] -> w472 mode=concatenating
                        tunnel: [w479] -> w471
                        tunnel: w470 -> [w477]
                        tunnel: w469 -> [w478]
                        tunnel: [w478] -> w466
                        tunnel: [w477] -> w463
                        tunnel: [w475] -> w468 mode=concatenating
                        n125 = Unbundle(w483) -> ("Array of fetched data"=w482:dbl[][][], "Channel Names Array"=w481:string[])  [unwired: 4 out]
                        n126 = Index Array(array=w482, index (dim 0)=w480) -> (element=w476:dbl[][])  [unwired: 2 in]
                        n127 = Index Array(array=w481, index=w480) -> (element=w479:string)
                        n128 = Array Size(array=w476) -> (size(s)=w475:i32[])
                      }
                      n129 = Bundle("Array of fetched data"=w472, w471, w468) -> (w467:T3)  [unwired: 1 in]
                      "data going into the binary file" <- w467
                      n130 = call "DataFileNode_Entry_V4.vi"("error in (no error)"=w465, "Queued Elements"=w467, "Byte Stream File in"=w466) -> ("error out"=w462:errorcluster, "Byte Stream File out"=w464:refnum<file>)  [unwired: 7 in]
                    }
                  }
                }
              }
            }
          }
        }
        n131 = local read "Exiting"() -> (w336:bool)
        n132 = Equal To 0?(x=w337) -> (x = 0?=w335:bool)
        n133 = And(x=w335, y=w336) -> (x .and. y?=w334:bool)
      }
      "DCPowerInformationClusterArray_Input 2" <- w324
    }
    frame Disabled {
    }
  }
  n134 = for {
    tunnel: w7 -> [w488] mode=indexing
    tunnel: w6 -> [w486] mode=indexing
    shift-right: [w484] -> w4
    shift-left: w5 -> [w487]
    n135 = Close File(refnum=w488, error in=w487) -> (error out=w485:errorcluster)  [unwired: 1 out]
    n136 = Close File(refnum=w486, error in=w485) -> (error out=w484:errorcluster)  [unwired: 1 out]
  }
  n137 = Merge Errors(w10, w4) -> (w3:errorcluster)
  n138 = disable-structure shown="Enabled" {
    disable-tunnel: w3 -> [w506 w555]
    disable-tunnel: w2 -> [w503 w556]
    disable-tunnel: [w489 w538] -> w1
    frame Disabled {
      w490 = 24
      (unwired) T4[] []
      # "structure where the instruments channels are all read in one file together"
      # "number of data file nodes"
      # "To be removed once we only have one data file node and one supplemental data file node channel again soon"
      n139 = List Folder(path=w503, error in=w506) -> (path out=w498:path, filenames=w505:string[], error out=w497:errorcluster)  [unwired: 2 in, 1 out]
      n140 = Array Size(array=w505) -> (size(s)=w504:i32)
      n141 = Multiply(x=w490, y=2) -> (x*y=w500:i32)
      n142 = Divide(x=w504, y=w500) -> (x/y=w502:dbl)
      n143 = Decrement(x=w502) -> (x-1=w501:dbl)
      n144 = for {
        N: w501 -> [_]
        tunnel: w498 -> [w527]
        shift-right: [w523] -> w489
        shift-left: w497 -> [w525]
        tunnel: T4 {"Array of fetched data"=[], "Channel Names Array"=[], "Voltage Waveform Array"=[], "Current Waveform Array"=[], "Resetting Time"=timestamp(0 s since 1904-01-01), "Beam Logic"=0.0} ("DCPower Queue Data Double Array Format") -> [w514]
        tunnel: [w508] -> w491 mode=concatenating
        tunnel: [w508] -> w495 mode=indexing
        tunnel: [w511] -> w494 mode=indexing
        tunnel: [w511] -> w493 mode=concatenating
        tunnel: 0 ("size(s)") -> [w510]
        tunnel: w490 -> [w509]
        i -> [w534]
        w515 = T16."open" ("operation (0:open)")
        w532 = "NULL0_part_"
        # "Will need to change the naming conventions for this"
        n145 = Increment(x=w534) -> (x+1=w535:i32)
        n146 = Number To Decimal String(number=w535) -> (decimal integer string=w531:string)  [unwired: 1 in]
        n147 = Concatenate Strings(w532, w531, "_datafile.bin") -> (w529:string)
        n148 = Concatenate Strings(w532, w531, "_supplementaldatanode.bin") -> (w528:string)
        n149 = Build Path(base path=w527, name or relative path=w529) -> (appended path=w526:path)
        n150 = Build Path(base path=w527, name or relative path=w528) -> (appended path=w524:path)
        n151 = Open/Create/Replace File(file path (use dialog)=w526, error in=w525, operation (0:open)=w515) -> (refnum out=w518:refnum<file>, error out=w519:errorcluster)  [unwired: 3 in, 1 out]
        n152 = Read from Binary File(5:w514, 8:w519, 9:T15."native, host order" ("byte order (0:big-endian, network order)"), 10:-1 ("count (1)"), 11:w518) -> (0:w520:errorcluster, 2:w508:T4[])  [unwired: 1 in, 2 out]
        "datafile in loop" <- w508
        n153 = Open/Create/Replace File(file path (use dialog)=w524, error in=w520, operation (0:open)=w515) -> (refnum out=w521:refnum<file>, error out=w522:errorcluster)  [unwired: 3 in, 1 out]
        n154 = Read from Binary File(5:w510, 8:w522, 9:T15."native, host order" ("byte order (0:big-endian, network order)"), 10:-1 ("count (1)"), 11:w521) -> (0:w523:errorcluster, 2:w511:i32[])  [unwired: 1 in, 2 out]
        "supplemental datafile" <- w511
        n155 = for {
          tunnel: w508 -> [w536]
          i -> [w537]
          n156 = Index Array(array=w536, index=w537) -> ()  [unwired: 1 out]
        }
      }
      "datafile in concatenation" <- w491
      "datafile in array" <- w495
      "supplemental datafile array" <- w494
      "supplemental datafile concatenated" <- w493
      n157 = for {
        tunnel: w491 -> [w507] mode=indexing
      }
    }
    frame Enabled {
      # "number of bin files"
      # "datafile and supplemental parameters file"
      # "for now it will be 24 since we're using all channells of a 4163"
      # "NEED DATA PARAMETERS FILE TO KNOW HOW MANY DC POWER LOGS WERE RECORDED TO ACCURATELY PARSE THIS"
      n158 = List Folder(path=w556, error in=w555) -> (path out=w544:path, filenames=w554:string[], error out=w547:errorcluster)  [unwired: 2 in, 1 out]
      n159 = Array Size(array=w554) -> (size(s)=w553:i32)
      n160 = Multiply(x=24.0, y=2.0) -> (x*y=w550:dbl)
      n161 = Divide(x=w553, y=w550) -> (x/y=w548:dbl)
      n162 = for {
        tunnel: w544 -> [w585]
        tunnel: string[] ["NULL0", "NULL1", "NULL2", "NULL3", "NULL4", "NULL5", "NULL6", "NULL7", "NULL8", "NULL9", "NULL10", "NULL11", "NULL12", "NULL13", "NULL14", "NULL15", "NULL16", "NULL17", "NULL18", "NULL19", "NULL20", "NULL21", "NULL22", "NULL23"] -> [w586] mode=indexing
        tunnel: w548 -> [w582]
        shift-right: [w584] -> w543
        shift-left: w547 -> [w583]
        tunnel: T3 {"Array of fetched data"=[], "", []} ("output cluster") -> [w581]
        tunnel: [w580] -> w545 mode=indexing
        n163 = for {
          N: w582 -> [_]
          tunnel: w586 -> [w606]
          tunnel: w585 -> [w599]
          shift-right: [w595] -> w584
          shift-left: w583 -> [w598]
          tunnel: w581 -> [w597]
          tunnel: [w593] -> w580 mode=concatenating
          i -> [w605]
          n164 = Number To Decimal String(number=w605) -> (decimal integer string=w608:string)  [unwired: 1 in]
          n165 = Concatenate Strings(w606, "_part_" ("string"), w608, "_datafile.bin" ("string")) -> (w600:string)
          n166 = Build Path(base path=w599, name or relative path=w600) -> (appended path=w602:path)
          n167 = Open/Create/Replace File(file path (use dialog)=w602, error in=w598, operation (0:open)=T16."open", access (0:read/write)=enum16{"read/write", "read-only", "write-only"}."read/write") -> (refnum out=w591:refnum<file>, error out=w592:errorcluster)  [unwired: 2 in, 1 out]
          n168 = Set File Position(refnum=w591, error in=w592) -> (refnum out=w590:refnum<file>, error out=w589:errorcluster)  [unwired: 2 in]
          n169 = Read from Binary File(5:w597, 8:w589, 9:T15."native, host order" ("byte order (0:big-endian, network order)"), 10:-1 ("count (1)"), 11:w590) -> (0:w596:errorcluster, 2:w593:T2, 3:w594:refnum<file>)  [unwired: 1 in, 1 out]
          "data iterating in loop" <- w593
          n170 = Close File(refnum=w594, error in=w596) -> (error out=w595:errorcluster)  [unwired: 1 out]
        }
        "each channel cluster" <- w580
      }
      "all channel clusters as a large array" <- w545
      n171 = for {
        tunnel: w545 -> [w575] mode=indexing
        tunnel: [w566] -> w542 mode=indexing
        tunnel: w544 -> [w570]
        shift-right: [w572] -> w539
        shift-left: w543 -> [w574]
        n172 = for {
          tunnel: w575 -> [w579] mode=indexing
          tunnel: [w578] -> w566 mode=concatenating
          shift-right: [w577] -> w573
          shift-left: w574 -> [w577]
          tunnel: [w576] -> w568 mode=indexing
          n173 = Unbundle(w579) -> ("Array of fetched data"=w578:dbl[][], w576:string)  [unwired: 1 out]
        }
        n174 = Concatenate Strings(w568, "_output.csv" ("string")) -> (w569:string)
        n175 = Build Path(base path=w570, name or relative path=w569) -> (appended path=w571:path)
        n176 = call-poly <vilib>:"Write Delimited Spreadsheet.vi"("file path (dialog if empty)"=w571, "2D data"=w566, "error in (no error)"=w573) -> ("error out"=w572:errorcluster)  [unwired: 11 in, 1 out]
      }
      n177 = for {
        tunnel: w542 -> [w560] mode=indexing
        shift-right: [w559] -> w540
        shift-left: dbl[][] [] ("Array of fetched data") -> [w561]
        shift-right: [w557] -> w538
        shift-left: w539 -> [w558]
        n178 = for {
          tunnel: w560 -> [w564] mode=indexing
          shift-right: [w563] -> w559
          shift-left: w561 -> [w565]
          shift-right: [w562] -> w557
          shift-left: w558 -> [w562]
          n179 = Insert Into Array(array=w565, new element=w564) -> (w563:dbl[][])  [unwired: 2 in]
        }
      }
      "Array of all channels?" <- w540
    }
  }
  "error out" <- w1
